vi "Implement Publication Policy.vi"(5 "Last Published Value":variant, 7 "Last Published Time":timestamp, 9 "New Value Time":timestamp, 10 "New Value":variant, 11 "IncrementValuePublication In":refnum<class "IncrementValuePublication.lvclass">) -> (0 "error out (Reject Publication)":errorcluster, 2 "Value to Publish":variant)   [LabVIEW 2017, in "PublicationPolicy.lvlib" / "IncrementValuePublication.lvclass"]
doc: "This method decides whether or not to send or otherwise handle the new data value. The policy is set and maintained by the subscriber. The Topic Actor knows no policy details, it just passes the new value in. If there is a failure inside this method, the Topic Actor must assume the listener is no longer valid (dead/unrecoverable) and should delete it from the Subscriber list.\n\n<License>\nCopyright © 2017 Composed Systems, LLC | All rights reserved\nwww.composed.io\n\nAuthor: Ethan Stern <ethan.stern@composed.io>\n\nThis software is provided \"AS IS\" WITHOUT WARRANTIES, either express or implied, AND IS FOR EDUCATIONAL PURPOSES ONLY.\n</License>"
uses:
  IncrementValuePublication.lvclass
  <vilib>/ErrorRing/Error Ring.xnode
  <vilib>/Utility/Data Type/NI_Data Type.lvlib
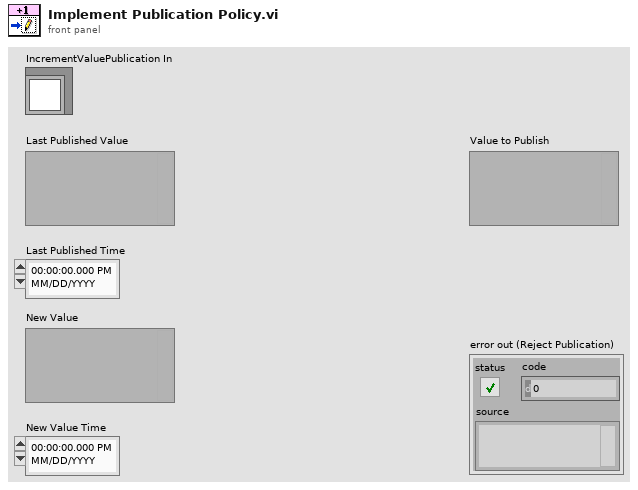
[diagram p1: front panel]
types:
  T1 = typedef "NI_Data Type.lvlib/Data Type.ctl" = enum8{"Invalid Type", "Void", "I8", "I16", "I32", "I64", "U8", "U16", "U32", "U64", "Single Float", "Double Float", "Extended Float", "Single Complex", "Double Complex", "Extended Complex", "Enum U8", "Enum U16", "Enum U32", "Enum U64", "Single Float With Unit", "Double Float With Unit", "Extended Float With Unit", "Single Complex with Unit", "Double Complex with Unit", "Extended Complex with Unit", "Boolean", "String", "Path", "Picture", "Tag", "Array", "Cluster", "Variant", "LV Variant", "Waveform", "Timestamp", "Digital Waveform", "Digital Data", "ExpressData", "Refnum", "External Data", "VI", "Poly VI", "LabVIEW Class Instance", "Fixed Point"}
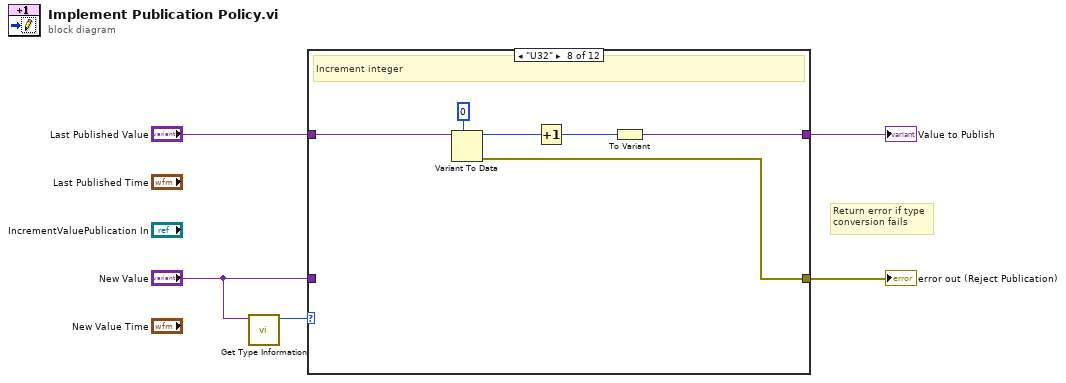
[diagram p0: block diagram]
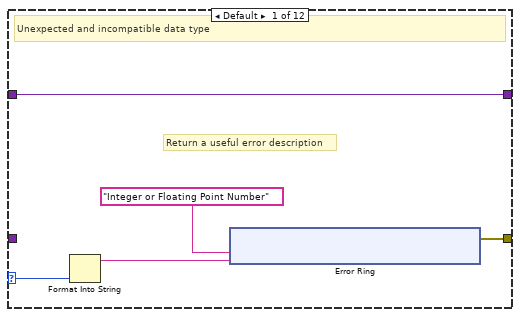
[diagram p2: hidden frame]
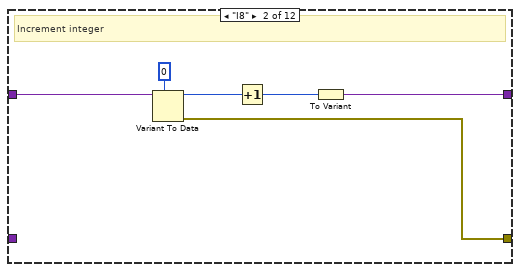
[diagram p3: hidden frame]
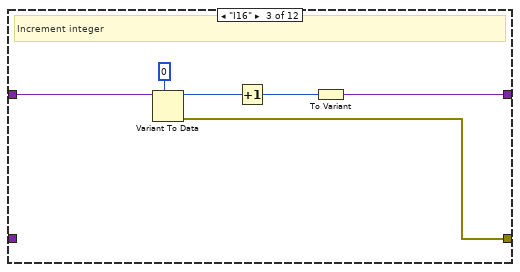
[diagram p4: hidden frame]
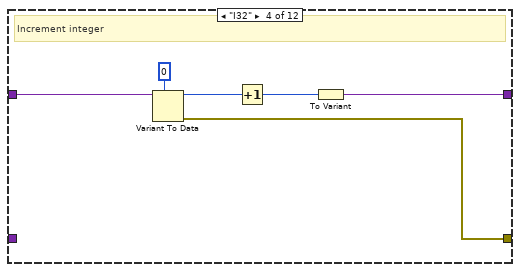
[diagram p5: hidden frame]
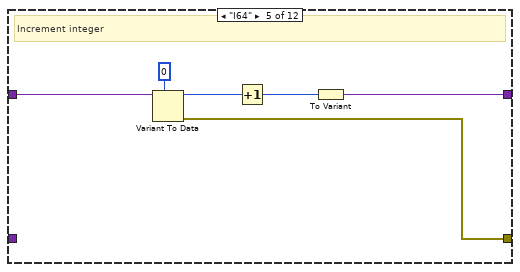
[diagram p6: hidden frame]
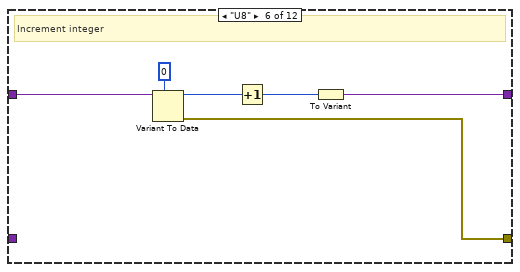
[diagram p7: hidden frame]
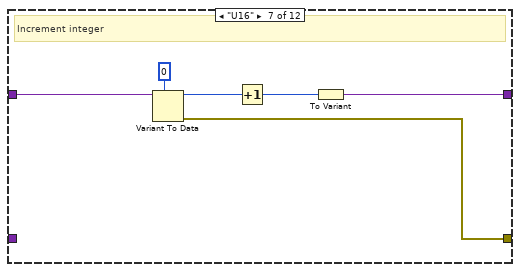
[diagram p8: hidden frame]
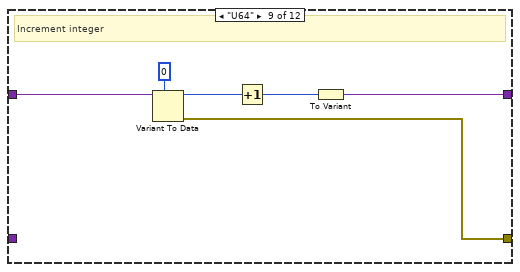
[diagram p9: hidden frame]
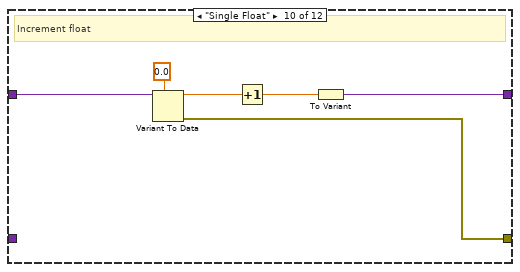
[diagram p10: hidden frame]
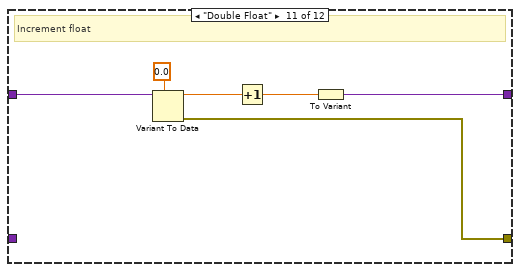
[diagram p11: hidden frame]
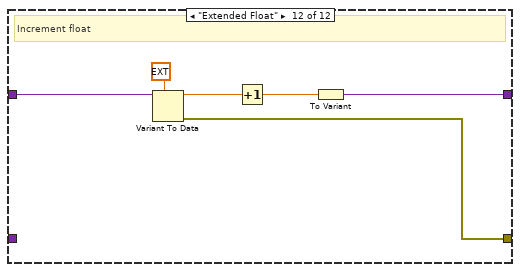
[diagram p12: hidden frame]
diagram:
  # "Return error if type\nconversion fails"
  n1 = call <vilib>:"Get Type Information.vi"("Variant"="New Value") -> ("Type"=w5:T1)  [unwired: 6 in, 4 out]
  n2 = case shown="\"U32\"" w5 {
    selector: w5 -> [w9 _ _ _ _ _ _ _ _ _ _ _]
    tunnel: "New Value" -> [_ _ _ _ _ _ _ _ _ _ _ _]
    tunnel: [w6 w21 w27 w33 w39 w45 w51 w57 w63 w67 w73 w79] -> w3
    tunnel: [w10 w20 w26 w32 w38 w44 w50 w56 w62 w66 w72 w78] -> w4
    tunnel: "Last Published Value" -> [w6 w18 w24 w30 w36 w42 w48 w54 w60 w70 w76 w82]
    frame Default {
      # "Return a useful error description"
      # "Unexpected and incompatible data type"
      n3 = Format Into String(w9) -> (resulting string=w8:string)  [unwired: 3 in, 1 out]
      n4 = xnode "Error Ring"("parameter 0"="Integer or Floating Point Number", "parameter 1"=w8) -> ("error out"=w10:errorcluster)
    }
    frame "I8" {
      # "Increment integer"
      n5 = Variant To Data(type=i8 0, Variant=w18) -> (data=w17:i8, error out=w20:errorcluster)  [unwired: 1 in]
      n6 = Increment(x=w17) -> (x+1=w19:i8)
      n7 = To Variant(anything=w19) -> (Variant=w21:variant)
    }
    frame "I16" {
      # "Increment integer"
      n8 = Variant To Data(type=i16 0, Variant=w24) -> (data=w23:i16, error out=w26:errorcluster)  [unwired: 1 in]
      n9 = Increment(x=w23) -> (x+1=w25:i16)
      n10 = To Variant(anything=w25) -> (Variant=w27:variant)
    }
    frame "I32" {
      # "Increment integer"
      n11 = Variant To Data(type=0, Variant=w30) -> (data=w29:i32, error out=w32:errorcluster)  [unwired: 1 in]
      n12 = Increment(x=w29) -> (x+1=w31:i32)
      n13 = To Variant(anything=w31) -> (Variant=w33:variant)
    }
    frame "I64" {
      # "Increment integer"
      n14 = Variant To Data(type=i64 0, Variant=w36) -> (data=w35:i64, error out=w38:errorcluster)  [unwired: 1 in]
      n15 = Increment(x=w35) -> (x+1=w37:i64)
      n16 = To Variant(anything=w37) -> (Variant=w39:variant)
    }
    frame "U8" {
      # "Increment integer"
      n17 = Variant To Data(type=u8 0, Variant=w42) -> (data=w41:u8, error out=w44:errorcluster)  [unwired: 1 in]
      n18 = Increment(x=w41) -> (x+1=w43:u8)
      n19 = To Variant(anything=w43) -> (Variant=w45:variant)
    }
    frame "U16" {
      # "Increment integer"
      n20 = Variant To Data(type=u16 0, Variant=w48) -> (data=w47:u16, error out=w50:errorcluster)  [unwired: 1 in]
      n21 = Increment(x=w47) -> (x+1=w49:u16)
      n22 = To Variant(anything=w49) -> (Variant=w51:variant)
    }
    frame "U32" {
      # "Increment integer"
      n23 = Variant To Data(type=u32 0, Variant=w54) -> (data=w53:u32, error out=w56:errorcluster)  [unwired: 1 in]
      n24 = Increment(x=w53) -> (x+1=w55:u32)
      n25 = To Variant(anything=w55) -> (Variant=w57:variant)
    }
    frame "U64" {
      # "Increment integer"
      n26 = Variant To Data(type=u64 0, Variant=w60) -> (data=w59:u64, error out=w62:errorcluster)  [unwired: 1 in]
      n27 = Increment(x=w59) -> (x+1=w61:u64)
      n28 = To Variant(anything=w61) -> (Variant=w63:variant)
    }
    frame "Single Float" {
      # "Increment float"
      n29 = Variant To Data(type=sgl 0.0, Variant=w70) -> (data=w69:sgl, error out=w66:errorcluster)  [unwired: 1 in]
      n30 = Increment(x=w69) -> (x+1=w65:sgl)
      n31 = To Variant(anything=w65) -> (Variant=w67:variant)
    }
    frame "Double Float" {
      # "Increment float"
      n32 = Variant To Data(type=0.0, Variant=w76) -> (data=w75:dbl, error out=w72:errorcluster)  [unwired: 1 in]
      n33 = Increment(x=w75) -> (x+1=w71:dbl)
      n34 = To Variant(anything=w71) -> (Variant=w73:variant)
    }
    frame "Extended Float" {
      # "Increment float"
      n35 = Variant To Data(type=ext 0.0, Variant=w82) -> (data=w81:ext, error out=w78:errorcluster)  [unwired: 1 in]
      n36 = Increment(x=w81) -> (x+1=w77:ext)
      n37 = To Variant(anything=w77) -> (Variant=w79:variant)
    }
  }
  "error out (Reject Publication)" <- w4
  "Value to Publish" <- w3
